vi "1.vi"() -> ()   [LabVIEW 2013]
panel:
  out "Minus":bool
  in  "X0":bool
  in  "X1":bool
  in  "X2":bool
  in  "X3":bool
  in  "X4":bool
  in  "X5":bool
  in  "X6":bool
  in  "X7":bool
  out "Boolean 15":bool
  out "Boolean 14":bool
  out "Boolean 13":bool
  out "Boolean 12":bool
  out "Boolean 11":bool
  out "Boolean 10":bool
  out "Boolean 9":bool
  out "Boolean 8":bool
  out "Boolean 7":bool
  out "Boolean 6":bool
  out "Boolean 5":bool
  out "Boolean 4":bool
  out "Boolean 3":bool
  out "Boolean 2":bool
  out "Boolean":bool
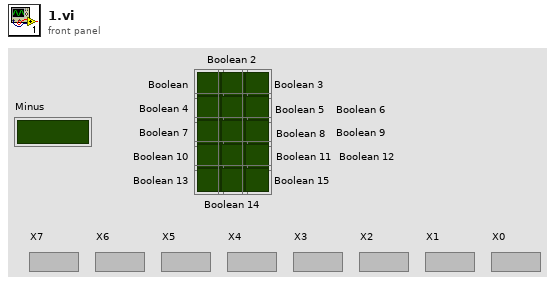
[diagram p1: front panel]
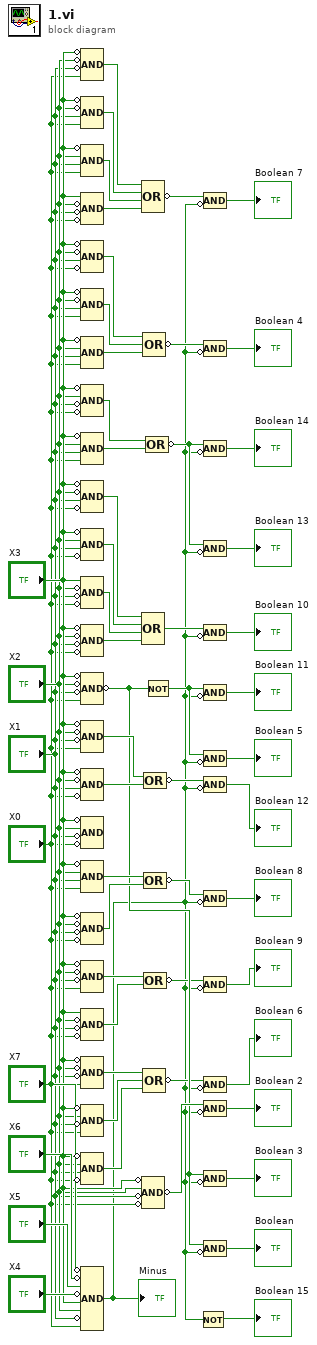
[diagram p0: block diagram]
diagram:
  n1 = Compound Arithmetic op=AND(invert "X3", invert "X2", invert "X1", "X0") -> (w37:bool)
  n2 = Compound Arithmetic op=AND(invert "X3", invert "X2", "X1", "X0") -> (w36:bool)
  n3 = Compound Arithmetic op=AND(invert "X3", "X2", "X1", "X0") -> (w51:bool)
  n4 = Compound Arithmetic op=AND("X3", invert "X2", invert "X1", invert "X0") -> (w50:bool)
  n5 = Compound Arithmetic op=AND(invert "X3", invert "X2", "X1", invert "X0") -> (w57:bool)
  n6 = Compound Arithmetic op=AND(invert "X3", invert "X2", "X1", "X0") -> (w56:bool)
  n7 = Compound Arithmetic op=AND(invert "X3", "X2", "X1", "X0") -> (w55:bool)
  n8 = Compound Arithmetic op=AND(invert "X3", "X2", invert "X1", invert "X0") -> (w40:bool)
  n9 = Compound Arithmetic op=AND(invert "X3", "X2", "X1", "X0") -> (w39:bool)
  n10 = Compound Arithmetic op=AND(invert "X3", invert "X2", "X1", invert "X0") -> (w46:bool)
  n11 = Compound Arithmetic op=AND(invert "X3", "X2", "X1", invert "X0") -> (w45:bool)
  n12 = Compound Arithmetic op=AND("X3", invert "X2", invert "X1", invert "X0") -> (w44:bool)
  n13 = Compound Arithmetic op=AND(invert "X3", invert "X2", invert "X1", invert "X0") -> (w43:bool)
  n14 = Compound Arithmetic op=AND(invert "X3", invert "X2", invert "X1", "X0") -> (invert w16:bool)
  n15 = Compound Arithmetic op=AND(invert "X3", invert "X2", invert "X1", "X0") -> (w42:bool)
  n16 = Compound Arithmetic op=AND(invert "X3", invert "X2", "X1", invert "X0") -> (w41:bool)
  n17 = Compound Arithmetic op=AND(invert "X3", "X2", invert "X1", invert "X0") -> ()  [unwired: 1 out]
  n18 = Compound Arithmetic op=AND(invert "X3", "X2", "X1", "X0") -> (w49:bool)
  n19 = Compound Arithmetic op=AND(invert "X3", invert "X2", invert "X1", invert "X0") -> (w48:bool)
  n20 = Compound Arithmetic op=AND(invert "X3", invert "X2", invert "X1", "X0") -> (w47:bool)
  n21 = Compound Arithmetic op=AND("X3", invert "X2", invert "X1", invert "X0") -> (w38:bool)
  n22 = Compound Arithmetic op=AND(invert "X3", invert "X2", invert "X1", "X0") -> (w54:bool)
  n23 = Compound Arithmetic op=AND(invert "X3", "X2", invert "X1", "X0") -> (w53:bool)
  n24 = Compound Arithmetic op=AND(invert "X3", "X2", "X1", invert "X0") -> (w52:bool)
  n25 = Compound Arithmetic op=AND(invert "X7", invert "X6", "X5", invert "X4", "X3", "X2", invert "X1", "X0") -> (w2:bool)
  "Minus" <- w2
  n26 = Compound Arithmetic op=OR(w37, w36, w51, w50) -> (invert w22:bool)
  n27 = Compound Arithmetic op=OR(w46, w45, w44, w43) -> (w12:bool)
  n28 = Compound Arithmetic op=AND(invert "X3", "X2", invert "X1", invert "X0") -> (invert w24:bool)
  n29 = Compound Arithmetic op=OR(w57, w56, w55) -> (invert w14:bool)
  n30 = Not(x=w16) -> (.not. x?=w19:bool)
  n31 = Compound Arithmetic op=OR(w54, w53, w52) -> (invert w4:bool)
  n32 = Compound Arithmetic op=OR(w42, w41) -> (invert w10:bool)
  n33 = Compound Arithmetic op=OR(w49, w48) -> (invert w8:bool)
  n34 = Compound Arithmetic op=OR(w47, w38) -> (invert w6:bool)
  n35 = Compound Arithmetic op=OR(w40, w39) -> (invert w26:bool)
  n36 = Not(x=w2) -> (.not. x?=→"Boolean 15":bool)
  n37 = Compound Arithmetic op=AND(w22, invert w2) -> (→"Boolean 7":bool)
  n38 = Compound Arithmetic op=AND(w14, invert w2) -> (→"Boolean 4":bool)
  n39 = Compound Arithmetic op=AND(w26, invert w2) -> (→"Boolean 14":bool)
  n40 = Compound Arithmetic op=AND(w26, invert w2) -> (→"Boolean 13":bool)
  n41 = Compound Arithmetic op=AND(w12, invert w2) -> (→"Boolean 10":bool)
  n42 = Compound Arithmetic op=AND(w19, invert w2) -> (→"Boolean 11":bool)
  n43 = Compound Arithmetic op=AND(w19, invert w2) -> (→"Boolean 5":bool)
  n44 = Compound Arithmetic op=AND(w10, invert w2) -> (→"Boolean 12":bool)
  n45 = Compound Arithmetic op=AND(w8, invert w2) -> (→"Boolean 8":bool)
  n46 = Compound Arithmetic op=AND(w6, invert w2) -> (→"Boolean 9":bool)
  n47 = Compound Arithmetic op=AND(w4, invert w2) -> (→"Boolean 6":bool)
  n48 = Compound Arithmetic op=AND(w24, invert w2) -> (→"Boolean 2":bool)
  n49 = Compound Arithmetic op=AND(w16, invert w2) -> (→"Boolean 3":bool)
  n50 = Compound Arithmetic op=AND(w16, invert w2) -> (→"Boolean":bool)
